vi "M04 Smart Grid try.vi"(9 "Target angle":sgl, 11 "EV3 in":T1) -> (3 "EV3 out":T1)   [LabVIEW 2016]
uses:
  <vilib>/NXT/Subs/LVHSConnector.ctl
  <vilib>/NXT/LegoClasses/BrickReference/BrickReference.lvclass
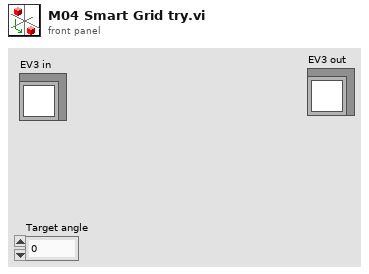
[diagram p1: front panel]
types:
  T1 = typedef "LVHSConnector.ctl" = refnum<class "BrickReference.lvclass">
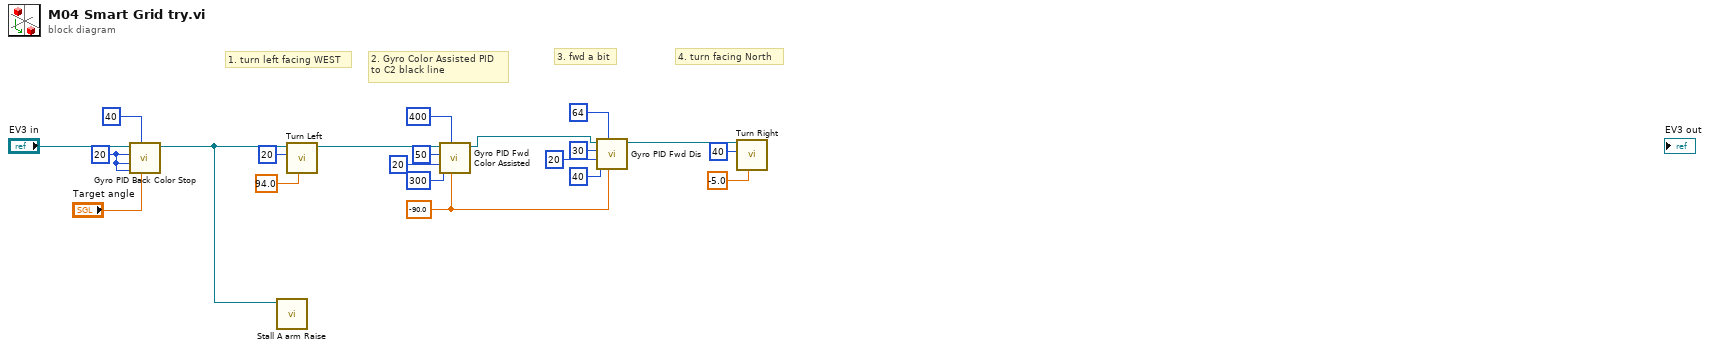
[diagram p0: block diagram]
diagram:
  w12 = 20 ("Max. speed")
  w1 = sgl -90.0 ("Target angle")
  # "4. turn facing North"
  # "3. fwd a bit"
  # "2. Gyro Color Assisted PID\nto C2 black line"
  # "1. turn left facing WEST"
  n1 = call "Gyro PID Back Color Stop.vi"("Target angle"="Target angle", "Threshold to Color"=40, "Threshold to slow"=w12, "Min. speed"=w12, "Max. speed"=w12, "EV3 in"="EV3 in") -> ("EV3 out"=w10:T1)  [unwired: 5 in]
  n2 = call "Stall A arm Raise.vi"("NXT/EV3"=w10) -> ()  [unwired: 10 in, 1 out]
  n3 = call "Turn Left.vi"("Turning angle"=sgl 94.0, "Motor B (right)"=i8 20, "EV3 in"=w10) -> ("EV3 out"=w15:T1)  [unwired: 8 in]
  n4 = call "Gyro PID Fwd Color Assisted.vi"("Target angle"=w1, "Threshold to Color"=400, "Threshold to slow"=300, "Min. speed"=20, "Max. speed"=50, "EV3 in"=w15) -> ("EV3 out"=w2:T1)  [unwired: 5 in]
  n5 = call "Gyro PID Fwd Dis.vi"("Target angle"=w1, "Threshold to stop"=64, "Threshold to slow"=40, "Min. speed"=20, "Max. speed"=30, "EV3 in"=w2) -> ("EV3 out"=w5:T1)  [unwired: 5 in]
  n6 = call "Turn Right.vi"("Turning angle"=sgl -5.0, "Motor B (right)"=i8 40, "EV3 in"=w5) -> ()  [unwired: 8 in, 1 out]
